vi "Assay to txt.vi"(11 "Array":string[](array[string])) -> (3 "String":string)   [LabVIEW 2013]
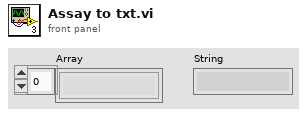
[diagram p1: front panel]
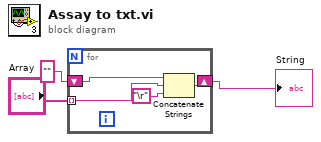
[diagram p0: block diagram]
diagram:
  n1 = for {
    tunnel: "Array" -> [w5] mode=indexing
    shift-right: [w7] -> w3
    shift-left: "" -> [w6]
    n2 = Concatenate Strings(w6, w5, "\r") -> (w7:string)
  }
  "String" <- w3
